vi "Untitled 3.vi"() -> ()   [LabVIEW 2020]
uses:
  <vilib>/Waveform/WDTOps.llb/WDT Get XY Value DBL.vi
panel:
  in  "stop":bool
  out "Pressure 2":dbl(graph)
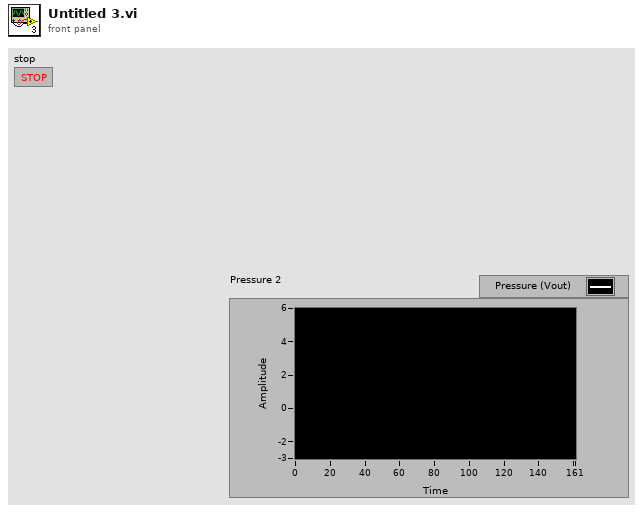
[diagram p1: front panel]
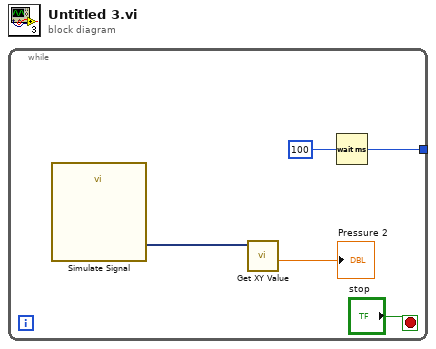
[diagram p0: block diagram]
diagram:
  n1 = while {
    tunnel: [w2] -> _
    stop <- "stop" stop-if-true
    n2 = call "Simulate Signal"() -> ("Sine"=w5:dynamicdata)  [unwired: 14 in, 1 out]
    n3 = call-poly <vilib>:"Get XY Value.vi"("waveform in"=w5) -> ("Y value"=→"Pressure 2":dbl)  [unwired: 6 in, 4 out]
    n4 = Wait (ms)(milliseconds to wait=u32 100) -> (millisecond timer value=w2:u32)
  }
